vi "Primary Viscosity.vi"(9 "Pri Cold Temp":dbl, 10 "Pri Hot Temp":dbl, 11 "Primary Average Temperature":dbl) -> (1 "FLiBe Viscosity (Pa-s) 2":dbl, 2 "FLiBe Viscosity (Pa-s) 3":dbl, 3 "FLiBe Ave Viscosity (Pa-s)":dbl, 4 "FLiBe Viscosity (Pa-s)":dbl, 5 "FLiBe Hot Viscosity (Pa-s)":dbl, 6 "FLiBe Cold Viscosity (Pa-s)":dbl)   [LabVIEW 2019]
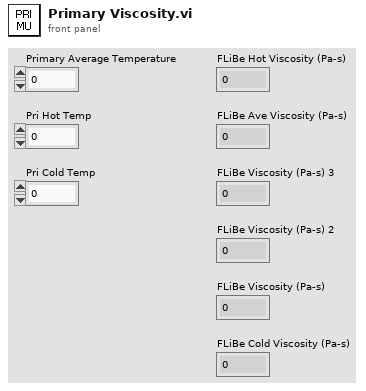
[diagram p1: front panel]
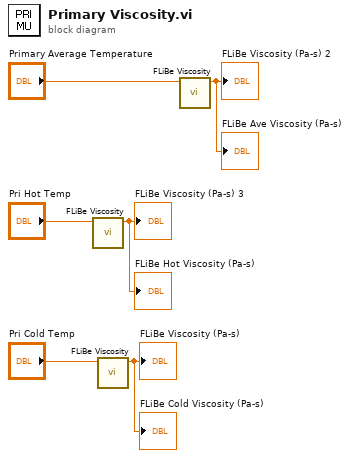
[diagram p0: block diagram]
diagram:
  n1 = call "FLiBe Viscosity.vi"("Temperature (K)"="Pri Hot Temp") -> ("FLiBe Viscosity (Pa-s)"=→"FLiBe Hot Viscosity (Pa-s)" →"FLiBe Viscosity (Pa-s) 3":dbl)  [unwired: 10 in]
  n2 = call "FLiBe Viscosity.vi"("Temperature (K)"="Pri Cold Temp") -> ("FLiBe Viscosity (Pa-s)"=→"FLiBe Cold Viscosity (Pa-s)" →"FLiBe Viscosity (Pa-s)":dbl)  [unwired: 10 in]
  n3 = call "FLiBe Viscosity.vi"("Temperature (K)"="Primary Average Temperature") -> ("FLiBe Viscosity (Pa-s)"=→"FLiBe Ave Viscosity (Pa-s)" →"FLiBe Viscosity (Pa-s) 2":dbl)  [unwired: 10 in]
